vi "Checkers How To Play.vi"() -> ()   [LabVIEW 2014]
panel:
  in  "Main Menu":bool
  # "HOW TO PLAY CHECKERS:"
  # "In checkers, each player starts out with 12 pieces. \nEach piece can move forward 1 space diagonally, to the \nleft or to the right (see left). (Player 1 moves up the board,\nand Player 2 moves down the board.) A piece can capture \n(remove) any opponent's piece/king by \"jumping\" over it, \nmoving forward 2 spaces diagonally over the enemy piece \n(see below)."
  # "A piece can't move onto a space already occupied by another piece/king. A player can't jump a piece over one of their own pieces (unless the own-man jumping  rule is enabled). Pieces can't move backwards. \n(See below.)"
  # "It's also possible for a piece to capture more than one\nof an opponent's pieces/kings in a single turn by \nmaking multiple forward jumps. A piece can change \ndirection mid-jump-combo, as long as it keeps\nmoving forward, never backward (see below)."
  # "X"
  # "X"
  # "X"
  # "X"
  # "X"
  # "X"
  # "When a player's piece reaches the opposite end \nof the board, the piece is \"promoted\" to a king.\nA player can have multiple king pieces. \n(See below left, below right.)"
  # "KING"
  # "A king piece can move and capture \nforwards or backwards!"
  # "KING"
  # "KING"
  # "KING"
  # "(A king faces similar move limitations\nas a piece: it can't share a space with another\nking/piece, and unless the own-man jump \nrule is enabled, also can't jump over its \nother pieces/kings of the same color.)"
  # "At the start of each game, each player starts off \nwith 12 pieces, arranged like so:"
  # "Player 1 moves first (because they're player 1).\nPlayers take alternating turns, moving 1 piece/king \nat a time as described above."
  # "There are 3 ways to win at checkers: \n1) Remove all your opponent's pieces from the board,\n2) Trap your opponent's pieces, so that your opponent\ncan't move any of their pieces/kings when it's their turn, or\n3) Get your opponent to surrender."
  # "-->Own-Man Jump Rule:\nYour pieces can hop over each other,\nincluding during multi-jump combos\n\n-->Force Capture Rule:\nIf your opponent moves a piece/king \nso that one of your pieces/kings\ncan capture it, you MUST capture it \non your turn."
  # "Additional Rules:"
  # "(Can be turned on and off in settings)"
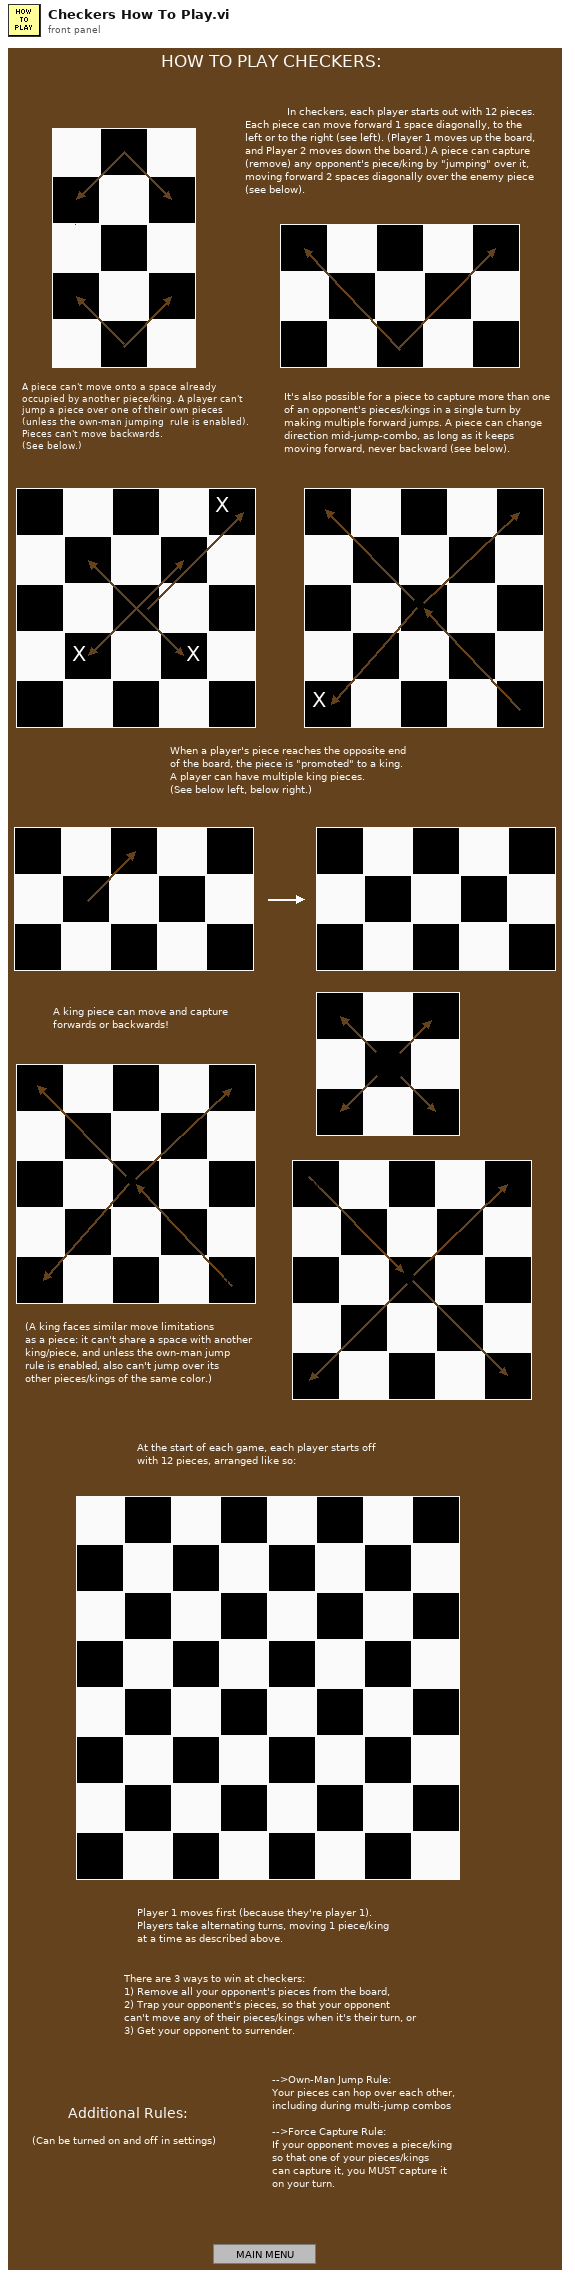
[diagram p1: front panel]
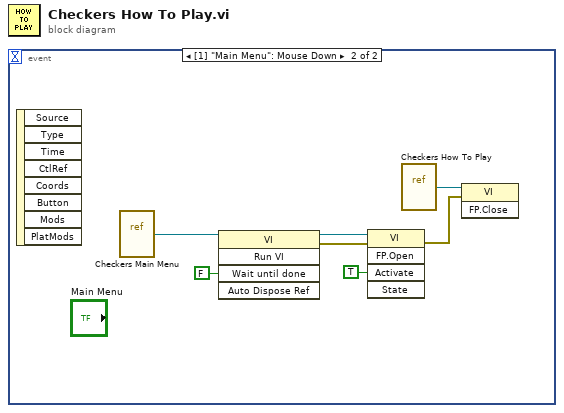
[diagram p0: block diagram]
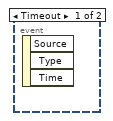
[diagram p2: hidden frame]
diagram:
  n1 = event shown="[1] \"Main Menu\": Mouse Down" {
    selector: _ -> [_ _]
    dyn-events: _ -> [_ _]
    timeout: _ -> [_ _]
    event Timeout {
      n2 = event-data() -> ()  [unwired: 1 in, 3 out]
    }
    event "Main Menu": Mouse Down {
      n3 = event-data() -> ()  [unwired: 1 in, 8 out]
      n4 = vi-ref "Checkers Main Menu.vi"() -> (w2:refnum<vi>)
      n5 = invoke class="VI" method="Run VI"(reference=w2, "Wait until done"=FALSE ("Wait Until Done")) -> (reference out=w3:refnum<vi>, error out=w4:errorcluster)  [unwired: 3 in, 3 out]
      n6 = invoke class="VI" method="FP.Open"(reference=w3, error in=w4, "Activate"=TRUE ("Activate?")) -> (error out=w7:errorcluster)  [unwired: 2 in, 4 out]
      n7 = vi-ref "Checkers How To Play.vi"() -> (w1:refnum<vi>)
      n8 = invoke class="VI" method="FP.Close"(reference=w1, error in=w7) -> ()  [unwired: 1 in, 3 out]
    }
  }
